vi "asynchronous background process.vi"(10 "async data in":T1, 11 "module runtime in":refnum<class "TBM module execution interface.lvclass">) -> (0 "error out":errorcluster, 3 "module runtime out":refnum<class "TBM module execution interface.lvclass">)   [LabVIEW 2013, in "Standard Engine Runtime.lvclass"]
uses:
  Standard Engine Runtime.lvclass
  asynchronous process data.ctl
  <vilib>/NI/Tag Bus Module Framework/runtime/TBM module execution interface.lvclass
  async command notification.ctl
  <vilib>/NI/Tag Bus/table/data table.ctl
  <vilib>/NI/Tag Bus Module Framework/runtime/execution settings.ctl
  async error info.ctl
  <vilib>/NI/Tag Bus Module Framework/runtime/error classification.ctl
  <vilib>/NI/Tag Bus/table/data table.lvlib
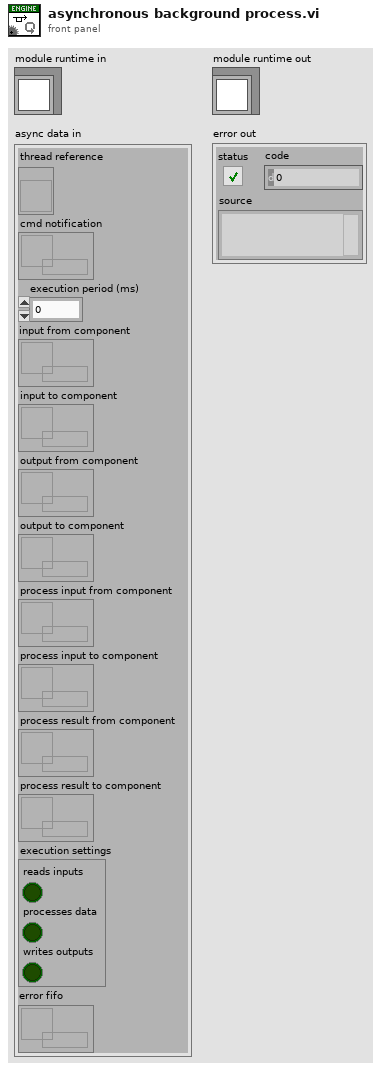
[diagram p1: front panel]
types:
  T1 = typedef "Standard Engine Runtime.lvclass/asynchronous process data.ctl" = cluster{"thread reference":refnum<vi>, "cmd notification":refnum<k33>, "execution period (ms)":i32, "input from component":refnum<queue>, "input to component":refnum<queue>, "output from component":refnum<queue>, "output to component":refnum<queue>, "process input from component":refnum<queue>, "process input to component":refnum<queue>, "process result from component":refnum<queue>, "process result to component":refnum<queue>, "execution settings":T2, "error fifo":refnum<k33>}
  T2 = typedef "TBM module execution interface.lvclass/execution settings.ctl" = cluster{"reads inputs":bool, "processes data":bool, "writes outputs":bool}
  T3 = typedef "TBM module execution interface.lvclass/error classification.ctl" = enum16{"unknown", "none", "trivial", "recoverable", "critical"}
  T4 = typedef "Standard Engine Runtime.lvclass/async error info.ctl" = cluster{"error code":i32, "error classification":T3}
  T5 = typedef "Standard Engine Runtime.lvclass/async command notification.ctl" = enum16{"stop", "safe state", "recover", "clear error"}
  T6 = typedef "tag bus.lvlib/data table.lvlib/data table.ctl" = cluster{"Double":dbl[], "Single":sgl[], "I64":i64[], "I32":i32[], "I16":i16[], "I8":i8[], "U64":u64[], "U32":u32[], "U16":u16[], "U8":u8[], "Boolean":bool[], "String":string[], "Array of Double":cluster{"DBL Array":dbl[]}[], "Array of Single":cluster{"SGL Array":sgl[]}[], "Array of I64":cluster{"I64 Array":i64[]}[], "Array of I32":cluster{"I32 Array":i32[]}[], "Array of I16":cluster{"I16 Array":i16[]}[], "Array of I8":cluster{"I8 Array":i8[]}[], "Array of U64":cluster{"U64 Array":u64[]}[], "Array of U32":cluster{"U32 Array":u32[]}[], "Array of U16":cluster{"U16 Array":u16[]}[], "Array of U8":cluster{"U8 Array":u8[]}[], "Array of Boolean":cluster{"Boolean Array":bool[]}[], "Array of String":cluster{"String Array":string[]}[]}
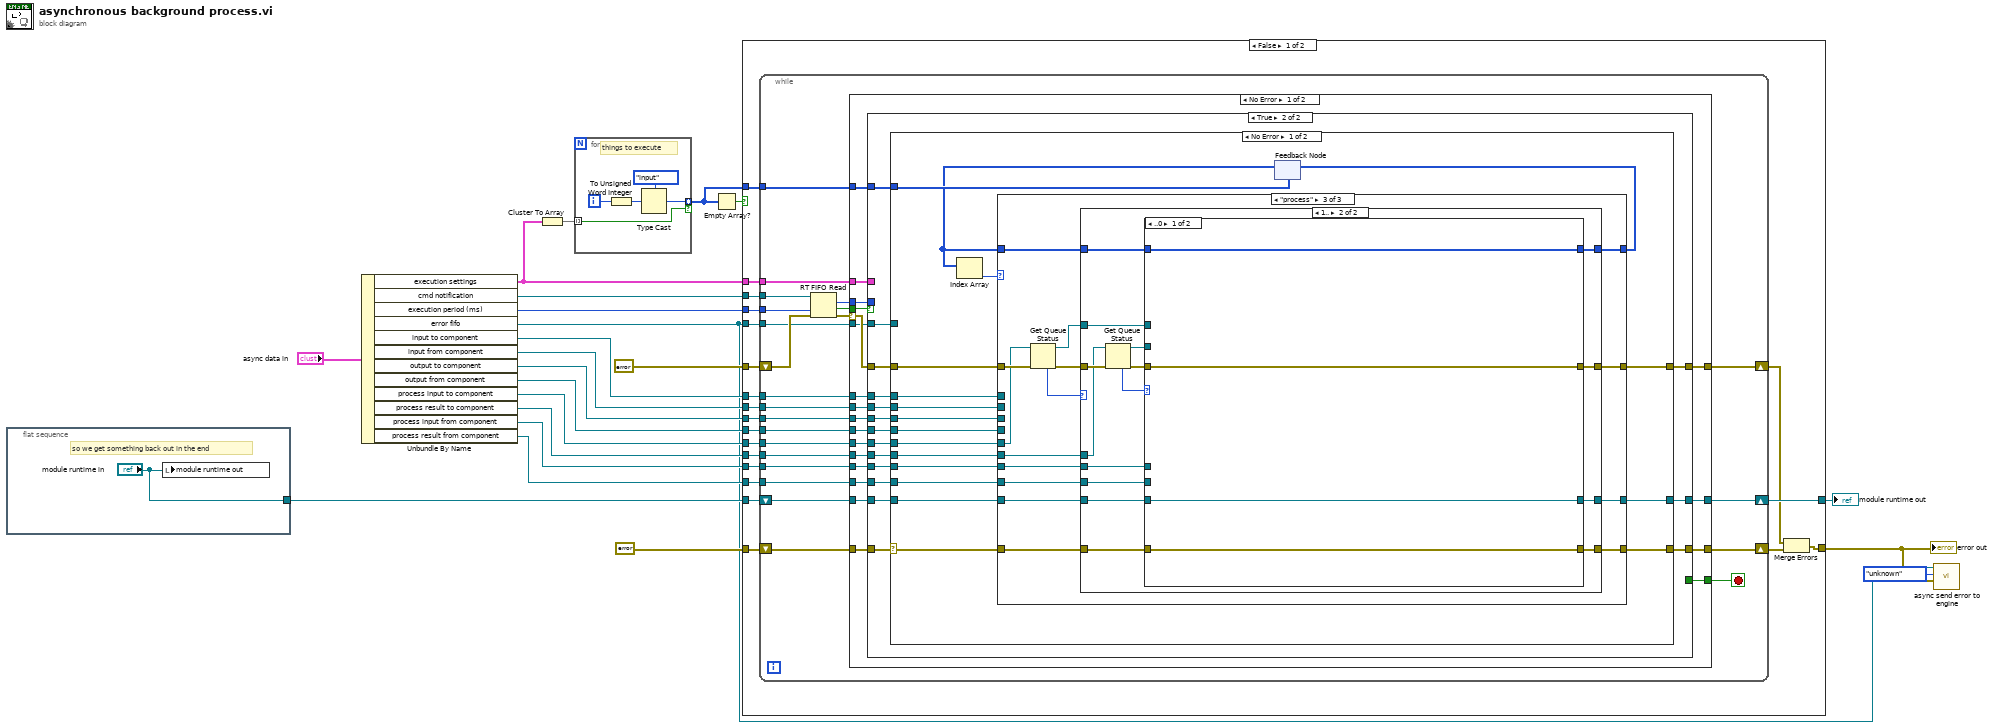
[diagram p0: block diagram]
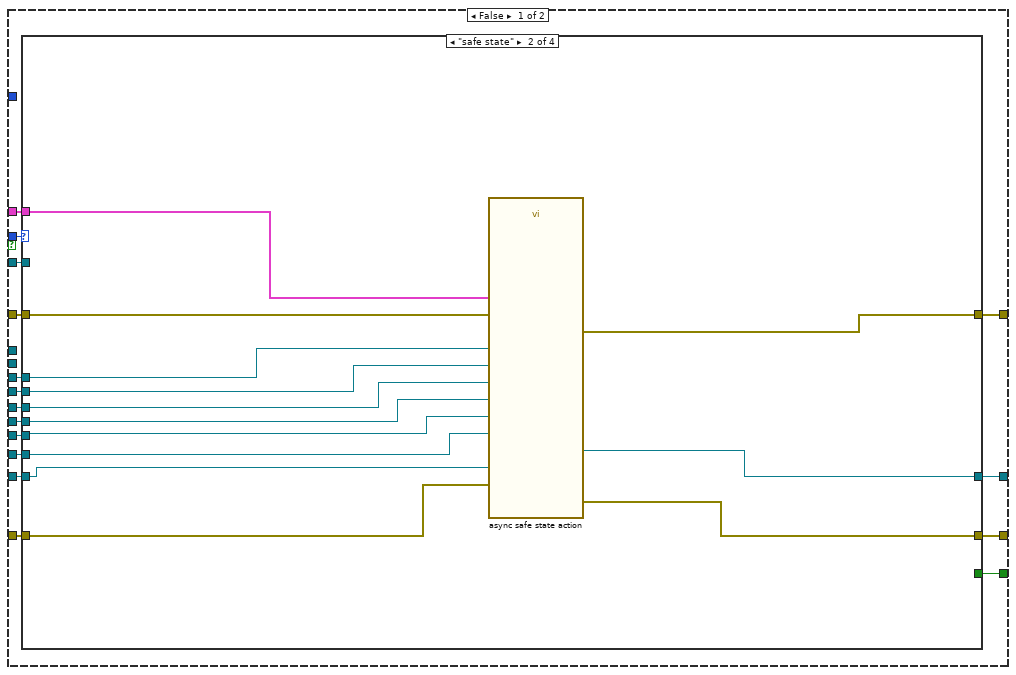
[diagram p2: hidden frame]
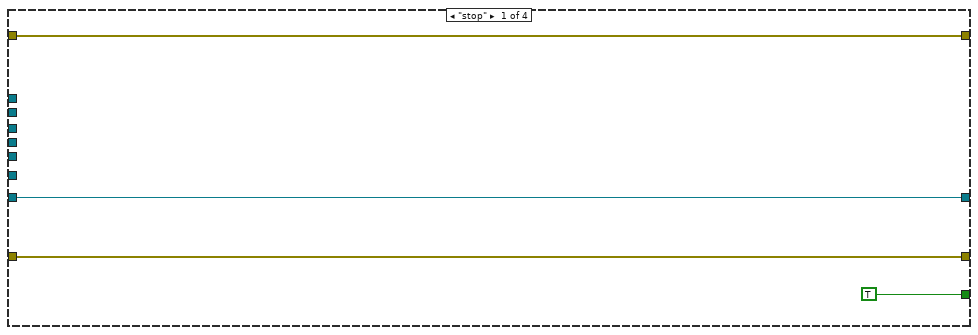
[diagram p3: hidden frame]
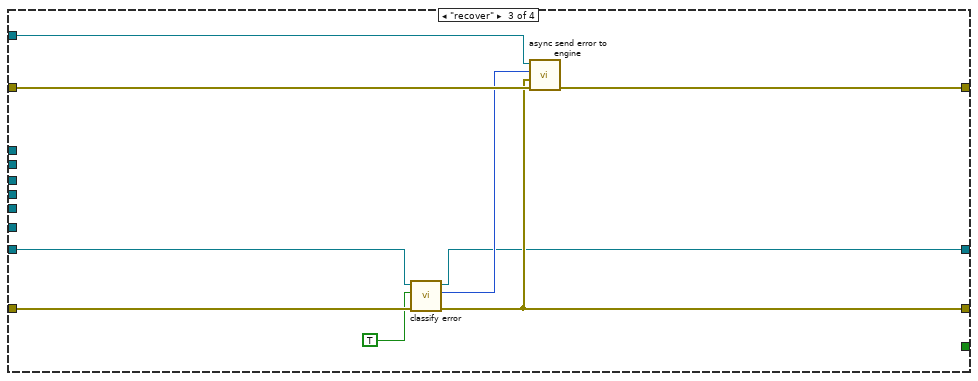
[diagram p4: hidden frame]
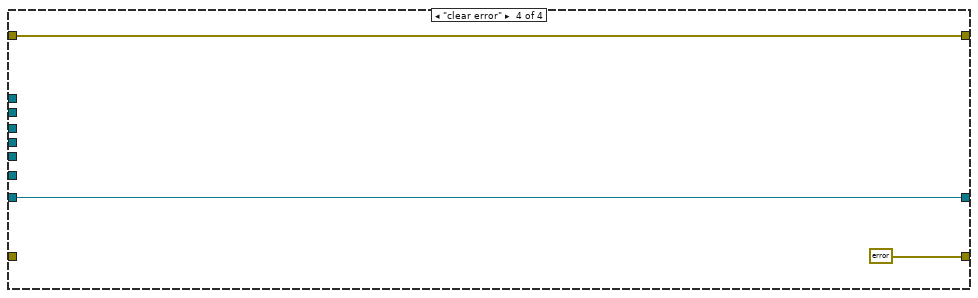
[diagram p5: hidden frame]
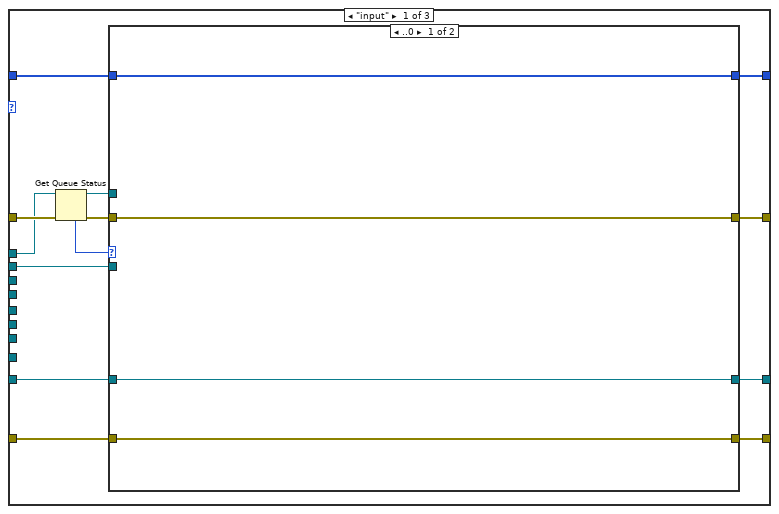
[diagram p6: hidden frame]
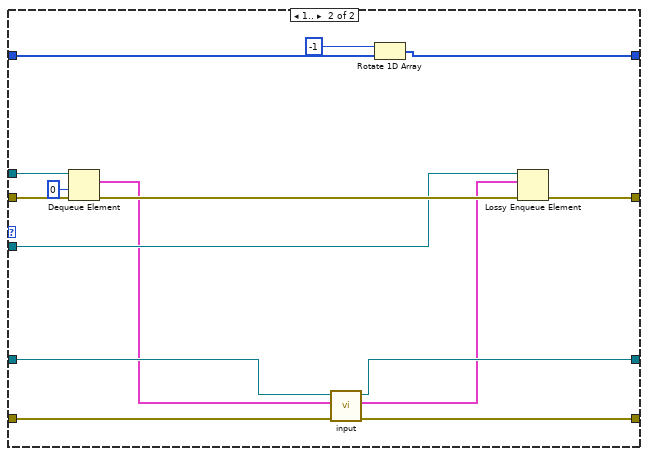
[diagram p7: hidden frame]
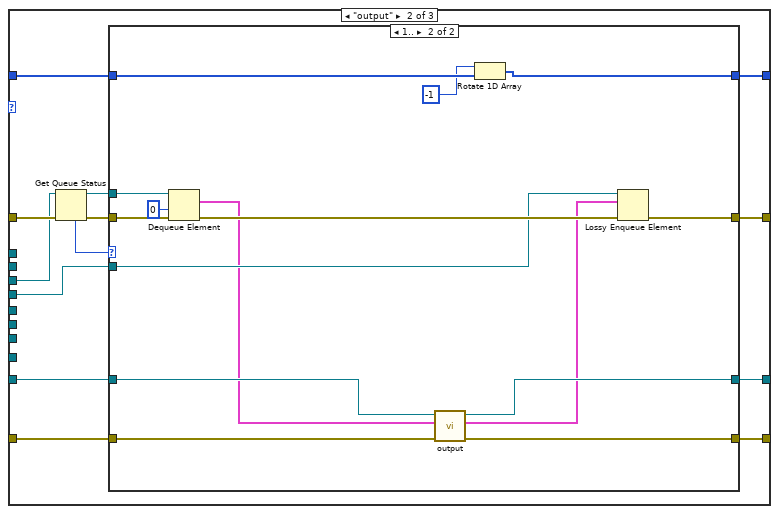
[diagram p8: hidden frame]
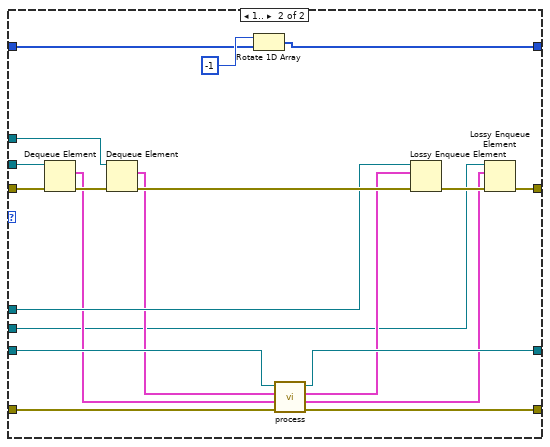
[diagram p11: hidden frame]
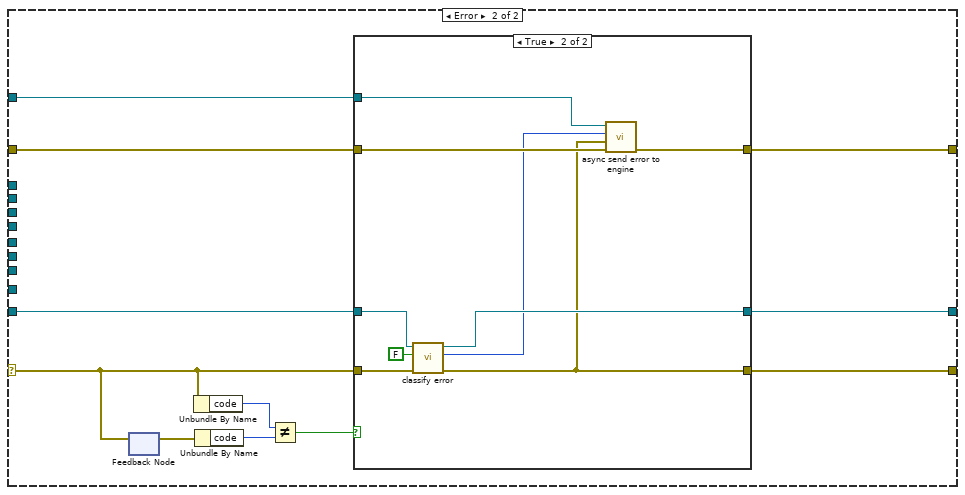
[diagram p12: hidden frame]
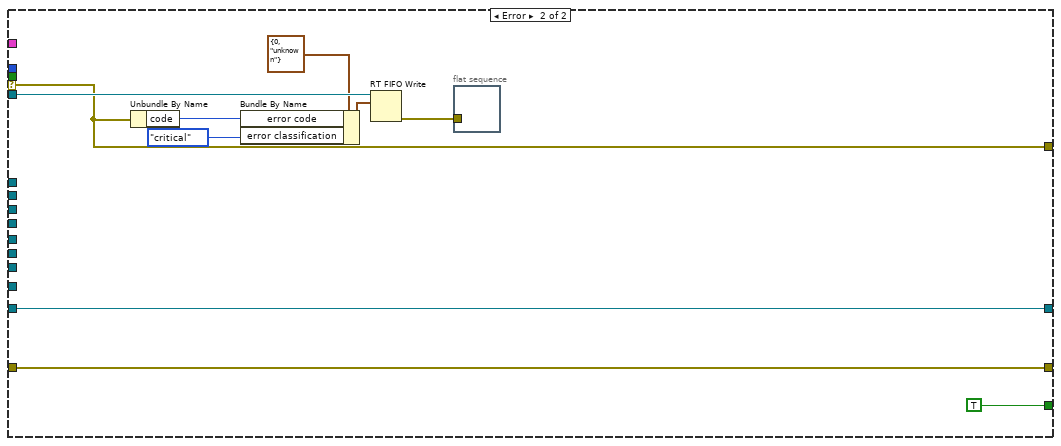
[diagram p14: hidden frame]
diagram:
  n1 = flat-sequence {
    tunnel: ["module runtime in"] -> w21
    frame #0 {
      # "so we get something back out in the end"
      n2 = local write "module runtime out"("module runtime in") -> ()
    }
  }
  n3 = Unbundle By Name("async data in") -> ("execution settings"=w1:T2, "cmd notification"=w19:refnum<k33>, "execution period (ms)"=w18:i32, "error fifo"=w4:refnum<k33>, "input to component"=w10:refnum<queue>, "input from component"=w9:refnum<queue>, "output to component"=w8:refnum<queue>, "output from component"=w11:refnum<queue>, "process input to component"=w12:refnum<queue>, "process result to component"=w13:refnum<queue>, "process input from component"=w14:refnum<queue>, "process result from component"=w15:refnum<queue>)
  n4 = Cluster To Array(cluster=w1) -> (array=w7:bool[])
  n5 = for {
    tunnel: w7 -> [w24] mode=indexing
    tunnel: [w25] -> w6 mode=indexing if=w24
    i -> [w26]
    # "things to execute"
    n6 = To Unsigned Word Integer(number=w26) -> (unsigned 16bit integer=w27:u16)
    n7 = Type Cast(type=enum16{"input", "process", "output"}."input" ("async execution state"), x=w27) -> (*(type *) &x=w25:enum16{"input", "process", "output"})
  }
  n8 = Empty Array?(array=w6) -> (empty?=w5:bool)
  n9 = case shown="False" w5 {
    tunnel: w21 -> [w48 w327]
    tunnel: [w47 w327] -> w20
    tunnel: w19 -> [w46 _]
    tunnel: w18 -> [w45 _]
    tunnel: errorcluster {"status"=FALSE, "code"=0, "source"=""} ("error out") -> [w44 w326]
    tunnel: [w41 w326] -> w3
    tunnel: w4 -> [w40 _]
    tunnel: errorcluster {"status"=FALSE, "code"=0, "source"=""} ("error out") -> [w39 _]
    tunnel: w15 -> [w38 _]
    tunnel: w14 -> [w37 _]
    tunnel: w13 -> [w36 _]
    tunnel: w12 -> [w35 _]
    tunnel: w11 -> [w34 _]
    tunnel: w10 -> [w33 _]
    tunnel: w9 -> [w32 _]
    tunnel: w8 -> [w31 _]
    tunnel: w6 -> [w30 _]
    tunnel: w1 -> [w29 _]
    frame False {
      n10 = while {
        shift-right: [w67] -> w47
        shift-left: w48 -> [w66]
        tunnel: w46 -> [w71]
        tunnel: w45 -> [w70]
        shift-right: [w64] -> w43
        shift-left: w44 -> [w63]
        shift-right: [w65] -> w42
        shift-left: w39 -> [w69]
        tunnel: w40 -> [w62]
        tunnel: w30 -> [w58]
        tunnel: w38 -> [w57]
        tunnel: w37 -> [w56]
        tunnel: w36 -> [w55]
        tunnel: w35 -> [w54]
        tunnel: w34 -> [w53]
        tunnel: w33 -> [w52]
        tunnel: w32 -> [w51]
        tunnel: w31 -> [w50]
        tunnel: w29 -> [w49]
        stop <- w61 stop-if-true
        n11 = RT FIFO Read(0:w71, 2:w70, 3:w69) -> (9:w60:T5, 10:w59:bool, 11:w68:errorcluster)  [unwired: 1 in, 2 out]
        n12 = case shown="No Error" w68 {
          selector: w68 -> [w86 w319]
          tunnel: [w88 w325] -> w67
          tunnel: w66 -> [w89 w325]
          tunnel: [w87 w319] -> w65
          tunnel: [w85 w324] -> w64
          tunnel: w63 -> [w73 w324]
          tunnel: w62 -> [w83 w323]
          tunnel: [w84 TRUE] -> w61
          tunnel: w60 -> [w90 _]
          tunnel: w59 -> [w91 _]
          tunnel: w58 -> [w82 _]
          tunnel: w57 -> [w81 _]
          tunnel: w56 -> [w80 _]
          tunnel: w55 -> [w79 _]
          tunnel: w54 -> [w78 _]
          tunnel: w53 -> [w77 _]
          tunnel: w52 -> [w76 _]
          tunnel: w51 -> [w75 _]
          tunnel: w50 -> [w74 _]
          tunnel: w49 -> [w72 _]
          frame No Error {
            n13 = case shown="True" w91 {
              tunnel: w90 -> [w107 _]
              tunnel: w89 -> [w106 w149]
              tunnel: [w105 w150] -> w88
              tunnel: [w104 w151] -> w87
              tunnel: w86 -> [w103 w152]
              tunnel: w73 -> [w102 w138]
              tunnel: [w101 w148] -> w85
              tunnel: [w100 _] -> w84
              tunnel: w83 -> [w99 w137]
              tunnel: w82 -> [_ w147]
              tunnel: w81 -> [w93 w146]
              tunnel: w80 -> [w94 w145]
              tunnel: w79 -> [w95 w144]
              tunnel: w78 -> [w96 w143]
              tunnel: w77 -> [w97 w142]
              tunnel: w76 -> [_ w141]
              tunnel: w75 -> [_ w140]
              tunnel: w74 -> [w98 w139]
              tunnel: w72 -> [w92 _]
              frame False {
                n14 = case shown="\"safe state\"" w107 {
                  tunnel: w106 -> [w111 w120 w125 w135]
                  tunnel: [w111 w119 w126 w135] -> w105
                  tunnel: [w110 w123 w130 w136] -> w104
                  tunnel: w103 -> [w110 w124 w131 w136]
                  tunnel: w102 -> [w109 w121 w133 _]
                  tunnel: [w109 w118 w127 errorcluster {"status"=FALSE, "code"=0, "source"=""} ("classified error")] -> w101
                  tunnel: [TRUE _ _ _] -> w100
                  tunnel: w99 -> [_ _ w129 _]
                  tunnel: w98 -> [_ w112 _ _]
                  tunnel: w97 -> [_ w113 _ _]
                  tunnel: w96 -> [_ w114 _ _]
                  tunnel: w95 -> [_ w115 _ _]
                  tunnel: w94 -> [_ w116 _ _]
                  tunnel: w93 -> [_ w117 _ _]
                  tunnel: w92 -> [_ w122 _ _]
                  frame "stop" {
                  }
                  frame "safe state" {
                    n15 = call "async safe state action.vi"("output to component"=w112, "system error in"=w124, "execution settings"=w122, "output from component"=w113, "process input to component"=w114, "process result to component"=w115, "process input from component"=w116, "process result from component"=w117, "module in"=w120, "module error in"=w121) -> ("system error out"=w123:errorcluster, "module out"=w119:refnum<class "TBM module execution interface.lvclass">, "module error out"=w118:errorcluster)  [unwired: 3 in]
                  }
                  frame "recover" {
                    n16 = call-dynamic "classify error.vi"("error to classify"=w133, "attempt recovery?"=TRUE, "module in"=w125) -> ("classified error"=w127:errorcluster, "error classification"=w128:T3, "module out"=w126:refnum<class "TBM module execution interface.lvclass">)  [unwired: 6 in]
                    n17 = call "async send error to engine.vi"("command error in"=w131, "module error"=w127, "error classification"=w128, "error fifo"=w129) -> ("command error out"=w130:errorcluster)  [unwired: 7 in]
                  }
                  frame "clear error" {
                  }
                }
              }
              frame True {
                n18 = case shown="No Error" w138 {
                  selector: w138 -> [w153 w297]
                  tunnel: w152 -> [w169 w303]
                  tunnel: [w168 w301] -> w151
                  tunnel: [w167 w300] -> w150
                  tunnel: w149 -> [w166 w299]
                  tunnel: [w165 w298] -> w148
                  tunnel: w147 -> [w164 _]
                  tunnel: w146 -> [w163 _]
                  tunnel: w145 -> [w162 _]
                  tunnel: w144 -> [w161 _]
                  tunnel: w143 -> [w160 _]
                  tunnel: w142 -> [w159 _]
                  tunnel: w141 -> [w158 _]
                  tunnel: w140 -> [w157 _]
                  tunnel: w139 -> [w156 _]
                  tunnel: w137 -> [_ w302]
                  frame No Error {
                    n19 = feedback #1(w164) -> (w154:enum16{"input", "process", "output"}[])
                    n20 = Index Array(array=w154) -> (element=w155:enum16{"input", "process", "output"})  [unwired: 1 in]
                    n21 = case shown="\"process\"" w155 {
                      tunnel: [w178 w211 w245] -> w170
                      tunnel: w169 -> [w183 w215 w249]
                      tunnel: [w177 w210 w244] -> w168
                      tunnel: [w176 w209 w243] -> w167
                      tunnel: w166 -> [w175 w208 w242]
                      tunnel: w153 -> [w174 w207 w241]
                      tunnel: [w173 w206 w240] -> w165
                      tunnel: w163 -> [_ _ w235]
                      tunnel: w162 -> [_ _ w236]
                      tunnel: w161 -> [_ _ w237]
                      tunnel: w160 -> [_ _ w238]
                      tunnel: w159 -> [_ w203 _]
                      tunnel: w158 -> [w182 _ _]
                      tunnel: w157 -> [w171 _ _]
                      tunnel: w156 -> [_ w204 _]
                      tunnel: w154 -> [w172 w205 w239]
                      frame "input" {
                        n22 = Get Queue Status(queue=w182, error in (no error)=w183) -> (queue out=w179:refnum<queue>, error out=w180:errorcluster, # elements in queue=w181:i32)  [unwired: 1 in, 5 out]
                        n23 = case shown="..0" w181 {
                          tunnel: w180 -> [w187 w201]
                          tunnel: w179 -> [_ w202]
                          tunnel: [w184 w191] -> w178
                          tunnel: [w187 w194] -> w177
                          tunnel: [w186 w196] -> w176
                          tunnel: w175 -> [w186 w198]
                          tunnel: w174 -> [w185 w199]
                          tunnel: [w185 w197] -> w173
                          tunnel: w172 -> [w184 w190]
                          tunnel: w171 -> [_ w193]
                          frame ..0 {
                          }
                          frame 1.. {
                            n24 = Dequeue Element(queue=w202, timeout in ms (-1)=0, error in (no error)=w201) -> (element=w192:T6, error out=w195:errorcluster)  [unwired: 2 out]
                            n25 = call-dynamic "input.vi"("error in"=w199, "input allocation"=w192, "module in"=w198) -> ("error out"=w197:errorcluster, "input data"=w189:T6, "module out"=w196:refnum<class "TBM module execution interface.lvclass">)  [unwired: 6 in]
                            n26 = Rotate 1D Array(1:w190, 2:-1 ("n")) -> (0:w191:enum16{"input", "process", "output"}[])
                            n27 = Lossy Enqueue Element(queue=w193, element=w189, error in (no error)=w195) -> (error out=w194:errorcluster)  [unwired: 3 out]
                          }
                        }
                      }
                      frame "output" {
                        n28 = Get Queue Status(queue=w204, error in (no error)=w215) -> (queue out=w212:refnum<queue>, error out=w213:errorcluster, # elements in queue=w214:i32)  [unwired: 1 in, 5 out]
                        n29 = case shown="1.." w214 {
                          tunnel: w213 -> [w219 w233]
                          tunnel: w212 -> [_ w234]
                          tunnel: [w216 w223] -> w211
                          tunnel: [w219 w226] -> w210
                          tunnel: [w218 w228] -> w209
                          tunnel: w208 -> [w218 w230]
                          tunnel: w207 -> [w217 w231]
                          tunnel: [w217 w229] -> w206
                          tunnel: w205 -> [w216 w222]
                          tunnel: w203 -> [_ w225]
                          frame ..0 {
                          }
                          frame 1.. {
                            n30 = Dequeue Element(queue=w234, timeout in ms (-1)=0, error in (no error)=w233) -> (element=w224:T6, error out=w227:errorcluster)  [unwired: 2 out]
                            n31 = call-dynamic "output.vi"("error in"=w231, "output data"=w224, "module in"=w230) -> ("error out"=w229:errorcluster, "output allocation"=w220:T6, "module out"=w228:refnum<class "TBM module execution interface.lvclass">)  [unwired: 6 in]
                            n32 = Rotate 1D Array(1:w222, 2:-1 ("n")) -> (0:w223:enum16{"input", "process", "output"}[])
                            n33 = Lossy Enqueue Element(queue=w225, element=w220, error in (no error)=w227) -> (error out=w226:errorcluster)  [unwired: 3 out]
                          }
                        }
                      }
                      frame "process" {
                        n34 = Get Queue Status(queue=w238, error in (no error)=w249) -> (queue out=w246:refnum<queue>, error out=w247:errorcluster, # elements in queue=w248:i32)  [unwired: 1 in, 5 out]
                        n35 = case shown="1.." w248 {
                          tunnel: w247 -> [w253 w268]
                          tunnel: w246 -> [_ w256]
                          tunnel: [w250 w264] -> w245
                          tunnel: [w253 w262] -> w244
                          tunnel: [w252 w259] -> w243
                          tunnel: w242 -> [w252 w260]
                          tunnel: w241 -> [w251 w258]
                          tunnel: [w251 w257] -> w240
                          tunnel: w239 -> [w250 w263]
                          tunnel: w237 -> [_ w267]
                          tunnel: w236 -> [_ w255]
                          tunnel: w235 -> [_ w254]
                          frame ..0 {
                          }
                          frame 1.. {
                            n36 = Get Queue Status(queue=w267, error in (no error)=w268) -> (queue out=w261:refnum<queue>, error out=w265:errorcluster, # elements in queue=w266:i32)  [unwired: 1 in, 5 out]
                            n37 = case shown="..0" w266 {
                              tunnel: w265 -> [w271 w292]
                              tunnel: [w272 w286] -> w264
                              tunnel: w263 -> [w272 w287]
                              tunnel: [w271 w285] -> w262
                              tunnel: w261 -> [_ w291]
                              tunnel: w260 -> [w270 w281]
                              tunnel: [w270 w280] -> w259
                              tunnel: w258 -> [w269 w282]
                              tunnel: [w269 w279] -> w257
                              tunnel: w256 -> [_ w289]
                              tunnel: w255 -> [_ w278]
                              tunnel: w254 -> [_ w274]
                              frame ..0 {
                              }
                              frame 1.. {
                                n38 = Dequeue Element(queue=w291, error in (no error)=w292) -> (element=w277:T6, error out=w290:errorcluster)  [unwired: 1 in, 2 out]
                                n39 = Dequeue Element(queue=w289, error in (no error)=w290) -> (element=w276:T6, error out=w283:errorcluster)  [unwired: 1 in, 2 out]
                                n40 = Rotate 1D Array(1:w287, 2:-1 ("n")) -> (0:w286:enum16{"input", "process", "output"}[])
                                n41 = call-dynamic "process.vi"("error in"=w282, "result allocation"=w277, "parameters"=w276, "module in"=w281) -> ("error out"=w279:errorcluster, "results"=w273:T6, "parameter allocation"=w275:T6, "module out"=w280:refnum<class "TBM module execution interface.lvclass">)  [unwired: 4 in]
                                n42 = Lossy Enqueue Element(queue=w278, element=w275, error in (no error)=w283) -> (error out=w284:errorcluster)  [unwired: 3 out]
                                n43 = Lossy Enqueue Element(queue=w274, element=w273, error in (no error)=w284) -> (error out=w285:errorcluster)  [unwired: 3 out]
                              }
                            }
                          }
                        }
                      }
                    }
                    n44 = feedback-in #1(w170) -> ()
                  }
                  frame Error {
                    n45 = feedback-in #2(w297) -> ()
                    n46 = feedback #2() -> (w296:errorcluster)  [unwired: 1 in]
                    n47 = Unbundle By Name(w297) -> ("code"=w294:i32)
                    n48 = Unbundle By Name(w296) -> ("code"=w295:i32)
                    n49 = Not Equal?(x=w294, y=w295) -> (x != y?=w293:bool)
                    n50 = case shown="True" w293 {
                      tunnel: w303 -> [w306 w315]
                      tunnel: w302 -> [_ w314]
                      tunnel: [w306 w313] -> w301
                      tunnel: [w305 w312] -> w300
                      tunnel: w299 -> [w305 w311]
                      tunnel: [w304 w308] -> w298
                      tunnel: w297 -> [w304 w307]
                      frame False {
                      }
                      frame True {
                        n51 = call-dynamic "classify error.vi"("error to classify"=w307, "attempt recovery?"=FALSE, "module in"=w311) -> ("classified error"=w308:errorcluster, "error classification"=w309:T3, "module out"=w312:refnum<class "TBM module execution interface.lvclass">)  [unwired: 6 in]
                        n52 = call "async send error to engine.vi"("command error in"=w315, "module error"=w308, "error classification"=w309, "error fifo"=w314) -> ("command error out"=w313:errorcluster)  [unwired: 7 in]
                      }
                    }
                  }
                }
              }
            }
          }
          frame Error {
            n53 = Unbundle By Name(w319) -> ("code"=w318:i32)
            n54 = Bundle By Name(cluster=T4 {"error code"=0, "error classification"=enum."unknown"} ("element"), "error code"=w318, "error classification"=error_classification."critical") -> (w320:T4)
            n55 = RT FIFO Write(0:w323, 1:w320) -> (11:w322:errorcluster)  [unwired: 3 in, 3 out]
            n56 = flat-sequence {
              tunnel: w322 -> [_]
              frame #0 {
              }
            }
          }
        }
      }
      n57 = Merge Errors(w42, w43) -> (w41:errorcluster)
    }
    frame True {
    }
  }
  "error out" <- w3
  "module runtime out" <- w20
  n58 = call "async send error to engine.vi"("module error"=w3, "error classification"=error_classification."unknown", "error fifo"=w4) -> ()  [unwired: 8 in, 1 out]
